vi "SpectralCentroid (SubVI).vi"(10 "Frequency Array":dbl[](array[numeric]), 11 "Positve Half of FFT with 0Hz and Nyquist":dbl[](array[numeric])) -> (2 "Sum of FFT Mags":dbl, 3 "Spectral Centroid":dbl)   [LabVIEW 2015]
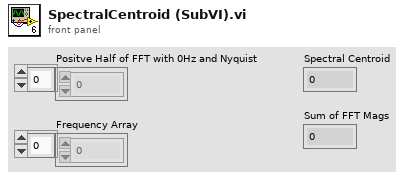
[diagram p1: front panel]
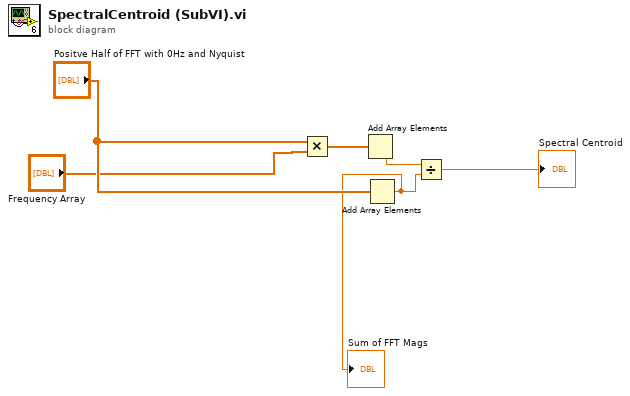
[diagram p0: block diagram]
diagram:
  n1 = Multiply(x="Positve Half of FFT with 0Hz and Nyquist", y="Frequency Array") -> (x*y=w2:dbl[])
  n2 = Add Array Elements(numeric array=w2) -> (sum=w1:dbl)
  n3 = Add Array Elements(numeric array="Positve Half of FFT with 0Hz and Nyquist") -> (sum=w5:dbl)
  "Sum of FFT Mags" <- w5
  n4 = Divide(x=w1, y=w5) -> (x/y=→"Spectral Centroid":dbl)
